vi "JSON to Status Tree.vi"(9 "JSON":string, 10 "Status Tree in":map{string[], T1}(c390)) -> (0 "error out":errorcluster, 2 "Status Tree":map{string[], T1}(c390))   [LabVIEW 2023, in "Volatus.lvlib" / "DebugHTTPController.lvclass"]
uses:
  DebugHTTPController.lvclass
  Module Status.ctl
  Module/State.ctl
  lv-cdm/CDM-Config/Config Element/Config Element.lvclass
  DebugHTTPController.lvclass/DebugHTTPController.ctl
  lv-cdm/CDM-Config/Config-JSON/Config-JSON.lvclass
  Module/Module.lvclass
  Volatus.lvlib
  lv-cdm/CDM-Config/Config Manager/Config Manager.lvclass
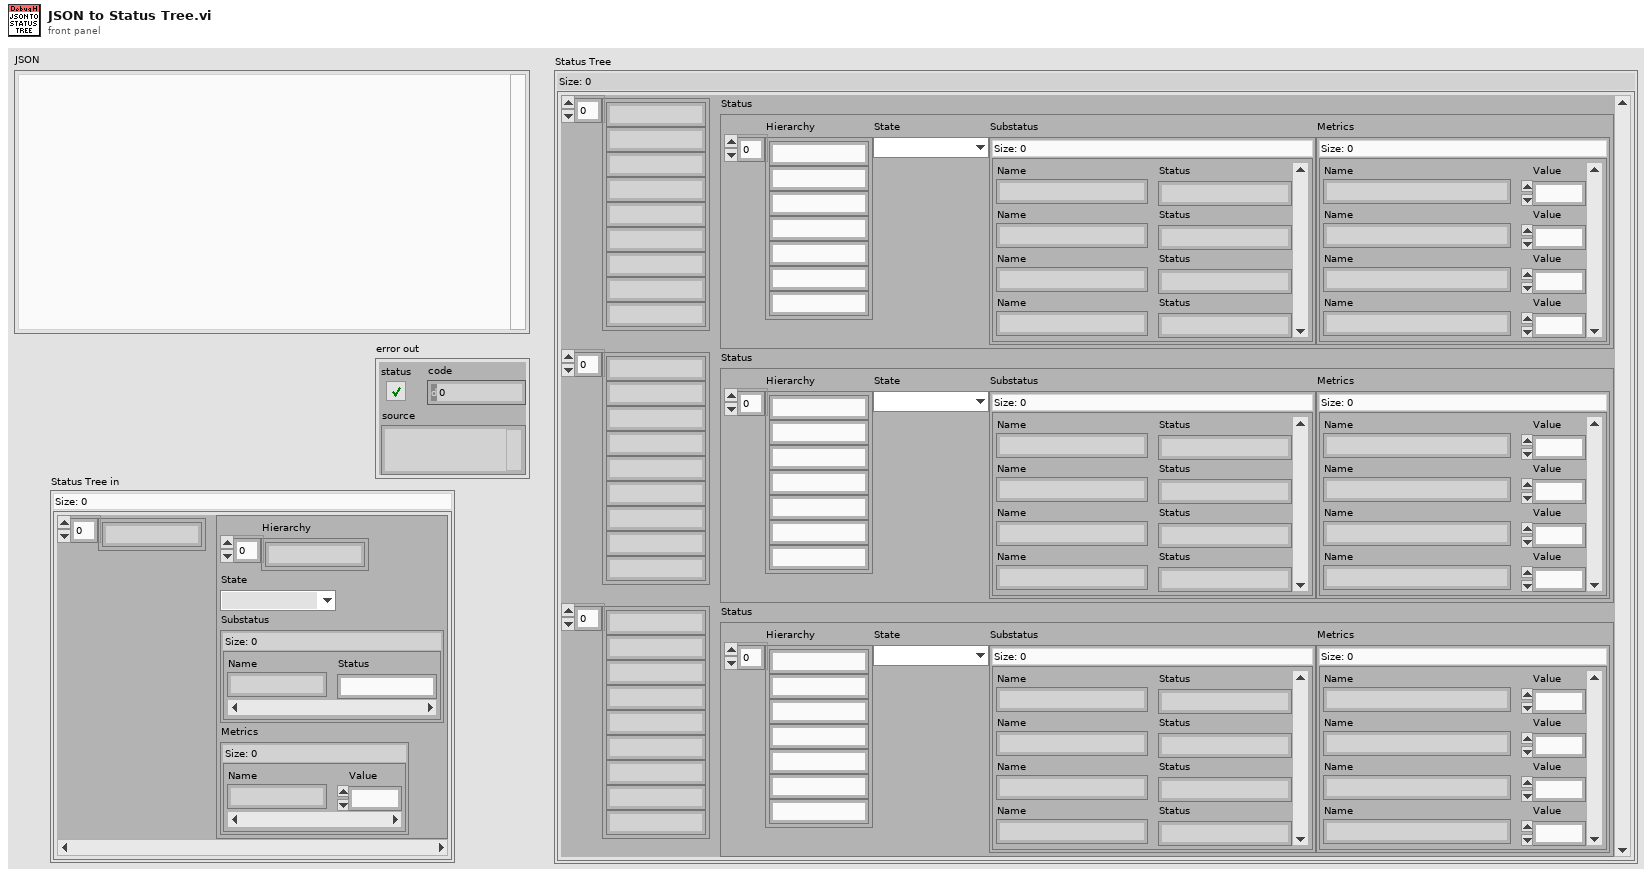
[diagram p1: front panel]
types:
  T1 = typedef "Volatus.lvlib/Module Status.ctl" = cluster{"Hierarchy":string[], "State":T2, "Substatus":map{string, string}, "Metrics":map{string, dbl}}
  T2 = typedef "Volatus.lvlib/Module.lvclass/State.ctl" = enum16{"Unknown", "Launched", "Starting", "Running", "Stopping", "Stopped", "Error - Starting", "Error - Run", "Error - Stopping"}
  T3 = cluster{"Parent":string[], "Element":refnum<class "Config Element.lvclass">}
  T4 = cluster{"Parent":string[], "Elements":refnum<class "Config Element.lvclass">}
  T5 = cluster{string[], "Elements":refnum<class "Config Element.lvclass">}
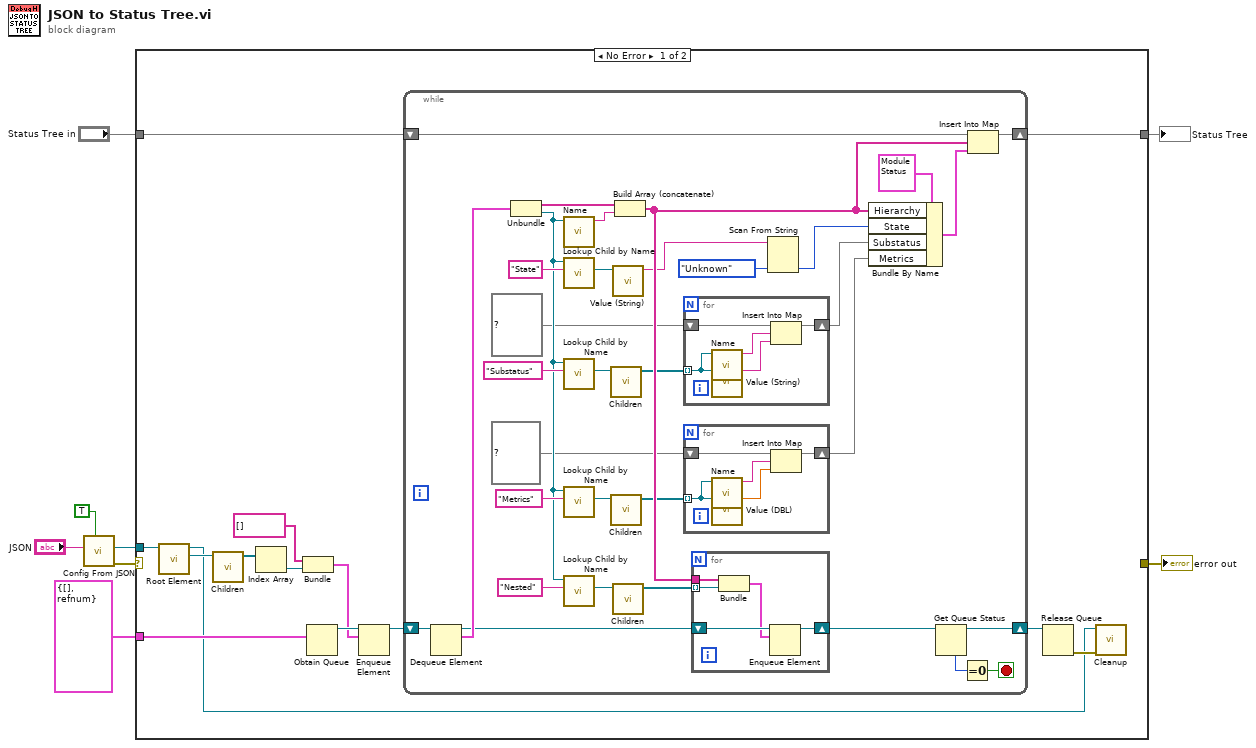
[diagram p0: block diagram]
diagram:
  n1 = call "Config From JSON.vi"("Mutable (F)"=TRUE, "JSON"="JSON") -> ("error out"=w7:errorcluster, "Config"=w6:refnum<class "Config Manager.lvclass">)  [unwired: 8 in]
  n2 = case shown="No Error" w7 {
    selector: w7 -> [_ w72]
    tunnel: w6 -> [w22 _]
    tunnel: T3 {"Parent"=[], "Element"=refnum} -> [w19 _]
    tunnel: [w13 w71] -> w4
    tunnel: [_ w72] -> w3
    tunnel: "Status Tree in" -> [w9 w71]
    frame No Error {
      n3 = call "Root Element.vi"("Config Manager in"=w22) -> ("Root Element"=w21:refnum<class "Config Element.lvclass">, "Config Manager out"=w10:refnum<class "Config Manager.lvclass">)  [unwired: 8 in, 1 out]
      n4 = call "Children.vi"("Config Element in"=w21) -> ("Elements"=w20:refnum<class "Config Element.lvclass">[])  [unwired: 9 in, 1 out]
      n5 = Index Array(array=w20) -> (element=w17:refnum<class "Config Element.lvclass">)  [unwired: 1 in]
      n6 = Bundle("Parent"=string[] [], "Elements"=w17) -> (w16:T4)  [unwired: 1 in]
      n7 = Obtain Queue(element data type=w19) -> (queue out=w18:refnum<queue>)  [unwired: 4 in, 2 out]
      n8 = Enqueue Element(queue=w18, element=w16) -> (queue out=w14:refnum<queue>)  [unwired: 2 in, 2 out]
      n9 = while {
        shift-right: [w50] -> w12
        shift-left: w14 -> [w55]
        shift-right: [w45] -> w13
        shift-left: w9 -> [w47]
        stop <- w48 stop-if-true
        n10 = Dequeue Element(queue=w55) -> (queue out=w38:refnum<queue>, element=w54:T3)  [unwired: 2 in, 2 out]
        n11 = Unbundle(w54) -> ("Parent"=w53:string[], "Element"=w40:refnum<class "Config Element.lvclass">)
        n12 = call "Name.vi"("Config Element in"=w40) -> ("Name"=w52:string)  [unwired: 9 in, 1 out]
        n13 = call "Lookup Child by Name.vi"("Name"="State", "Config Element in"=w40) -> ("Child"=w29:refnum<class "Config Element.lvclass">)  [unwired: 6 in, 3 out]
        n14 = call "Lookup Child by Name.vi"("Name"="Substatus", "Config Element in"=w40) -> ("Child"=w34:refnum<class "Config Element.lvclass">)  [unwired: 6 in, 3 out]
        n15 = call "Lookup Child by Name.vi"("Name"="Metrics", "Config Element in"=w40) -> ("Child"=w33:refnum<class "Config Element.lvclass">)  [unwired: 6 in, 3 out]
        n16 = call "Lookup Child by Name.vi"("Name"="Nested", "Config Element in"=w40) -> ("Child"=w39:refnum<class "Config Element.lvclass">)  [unwired: 6 in, 3 out]
        n17 = call "Children.vi"("Config Element in"=w34) -> ("Elements"=w32:refnum<class "Config Element.lvclass">[])  [unwired: 9 in, 1 out]
        n18 = call "Children.vi"("Config Element in"=w33) -> ("Elements"=w25:refnum<class "Config Element.lvclass">[])  [unwired: 9 in, 1 out]
        n19 = call "Value (String).vi"("Config Element in"=w29) -> ("String Value"=w23:string)  [unwired: 9 in, 1 out]
        n20 = call "Children.vi"("Config Element in"=w39) -> ("Elements"=w37:refnum<class "Config Element.lvclass">[])  [unwired: 9 in, 1 out]
        n21 = Build Array (concatenate)(w53, w52) -> (w36:string[])
        n22 = for {
          tunnel: w32 -> [w65] mode=indexing
          shift-right: [w61] -> w30
          shift-left: map{string, string} {} ("Substatus") -> [w64]
          n23 = call "Name.vi"("Config Element in"=w65) -> ("Name"=w63:string)  [unwired: 9 in, 1 out]
          n24 = call "Value (String).vi"("Config Element in"=w65) -> ("String Value"=w62:string)  [unwired: 9 in, 1 out]
          n25 = Insert Into Map(map in=w64, key=w63, value=w62) -> (map out=w61:map{string, string})  [unwired: 2 out]
        }
        n26 = for {
          tunnel: w25 -> [w60] mode=indexing
          shift-right: [w56] -> w24
          shift-left: map{string, dbl} {} ("Metrics") -> [w59]
          n27 = call "Name.vi"("Config Element in"=w60) -> ("Name"=w58:string)  [unwired: 9 in, 1 out]
          n28 = call "Value (DBL).vi"("Config Element in"=w60) -> ("DBL Value"=w57:dbl)  [unwired: 9 in, 1 out]
          n29 = Insert Into Map(map in=w59, key=w58, value=w57) -> (map out=w56:map{string, dbl})  [unwired: 2 out]
        }
        n30 = for {
          shift-right: [w66] -> w35
          shift-left: w38 -> [w68]
          tunnel: w37 -> [w70] mode=indexing
          tunnel: w36 -> [w69]
          n31 = Bundle(w69, "Elements"=w70) -> (w67:T5)  [unwired: 1 in]
          n32 = Enqueue Element(queue=w68, element=w67) -> (queue out=w66:refnum<queue>)  [unwired: 2 in, 2 out]
        }
        n33 = Scan From String(input string=w23, default 1=State."Unknown" ("State")) -> (output 1=w27:T2)  [unwired: 3 in, 3 out]
        n34 = Bundle By Name(cluster=T1 {"Hierarchy"=[], "State"=enum."Unknown", "Substatus"={}, "Metrics"={}} ("Module Status"), "Hierarchy"=w36, "State"=w27, "Substatus"=w30, "Metrics"=w24) -> (w46:T1)
        n35 = Get Queue Status(queue=w35) -> (queue out=w50:refnum<queue>, # elements in queue=w49:i32)  [unwired: 2 in, 6 out]
        n36 = Equal To 0?(x=w49) -> (x = 0?=w48:bool)
        n37 = Insert Into Map(map in=w47, key=w36, value=w46) -> (map out=w45:map{string[], T1})  [unwired: 2 out]
      }
      n38 = Release Queue(queue=w12) -> (error out=w11:errorcluster)  [unwired: 2 in, 2 out]
      n39 = call "Cleanup.vi"("error in (no error)"=w11, "Config Manager in"=w10) -> ()  [unwired: 9 in, 1 out]
    }
    frame Error {
    }
  }
  "Status Tree" <- w4
  "error out" <- w3
